vi "$TXXX.vi"(11 "反馈信息":string) -> (3 "接收信息":T1 {"校验和" format="%01xH"; "信息内容"."CRC标志" format="%01xH"; "信息内容"."发信时间分" format="%0d"; "信息内容"."发信时间时" format="%0d"; "信息内容"."信息类别" format="%01xH"})   [LabVIEW 2016, in "BD Protocol 4.0.lvlib" / "BD Protocol 4.0.lvclass"]
uses:
  BD Protocol 4.0.lvclass
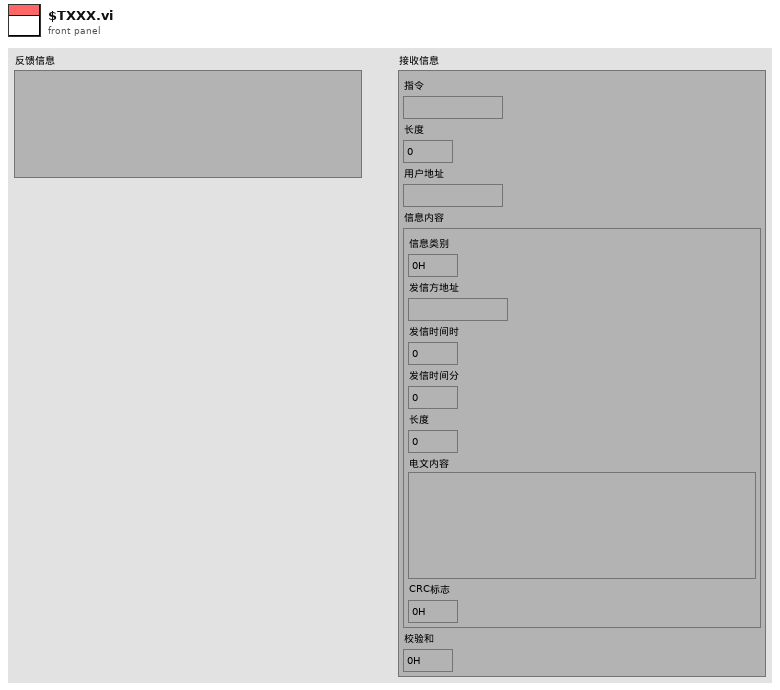
[diagram p1: front panel]
types:
  T1 = cluster{"指令":string, "长度":u16, "用户地址":string, "信息内容":cluster{"信息类别":u8, "发信方地址":string, "发信时间时":u8, "发信时间分":u8, "长度":u16, "电文内容":string, "CRC标志":u8}, "校验和":u8}
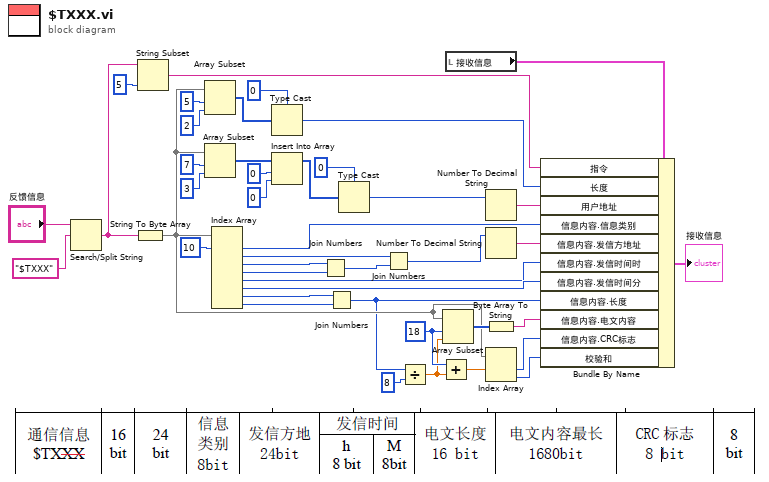
[diagram p0: block diagram]
diagram:
  w12 = 18 ("索引")
  n1 = Search/Split String(string="反馈信息", search string/char (-)="$TXXX" ("搜索字符串/字符(-)")) -> (match + rest of string=w39:string)  [unwired: 1 in, 2 out]
  n2 = String To Byte Array(string=w39) -> (unsigned byte array=w15:u8[])
  n3 = String Subset(string=w39, length (rest)=5 ("长度（剩余）")) -> (substring=w38:string)  [unwired: 1 in]
  n4 = Array Subset(array=w15, index=5 ("索引"), length=2 ("长度")) -> (w35:u8[])
  n5 = Array Subset(array=w15, index=7 ("索引"), length=3 ("长度")) -> (w30:u8[])
  n6 = Index Array(array=w15, index #1=10 ("索引")) -> (element #1=w23:u8, element #2=w18:u8, element #3=w20:u8, element #4=w21:u8, element #5=w4:u8, element #6=w5:u8, element #7=w6:u8, element #8=w7:u8)  [unwired: 7 in]
  n7 = Type Cast(type=u16 0 ("长度"), x=w35) -> (*(type *) &x=w33:u16)
  n8 = Insert Into Array(array=w30, index=0 ("索引"), new element=u8 0 ("新元素/子数组")) -> (w27:u8[])
  n9 = Join Numbers(hi=w20, lo=w21) -> ((hi.lo)=w19:u16)
  n10 = Join Numbers(hi=w6, lo=w7) -> ((hi.lo)=w13:u16)
  n11 = Type Cast(type=u32 0 ("长度"), x=w27) -> (*(type *) &x=w28:u32)
  n12 = Join Numbers(hi=w18, lo=w19) -> ((hi.lo)=w3:u32)
  n13 = Divide(x=w13, y=u16 8) -> (x/y=w8:dbl)
  n14 = Add(x=w12, y=w8) -> (x+y=w14:dbl)
  n15 = Array Subset(array=w15, index=w12, length=w8) -> (w17:u8[])
  n16 = local read "接收信息"() -> (w1:T1)
  n17 = Number To Decimal String(number=w28) -> (decimal integer string=w24:string)  [unwired: 1 in]
  n18 = Number To Decimal String(number=w3) -> (decimal integer string=w2:string)  [unwired: 1 in]
  n19 = Byte Array To String(unsigned byte array=w17) -> (string=w16:string)
  n20 = Index Array(array=w15, index #1=w14) -> (element #1=w11:u8, element #2=w10:u8)  [unwired: 1 in]
  n21 = Bundle By Name(cluster=w1, "指令"=w38, "长度"=w33, "用户地址"=w24, "信息内容.信息类别"=w23, "信息内容.发信方地址"=w2, "信息内容.发信时间时"=w4, "信息内容.发信时间分"=w5, "信息内容.长度"=w13, "信息内容.电文内容"=w16, "信息内容.CRC标志"=w11, "校验和"=w10) -> (→"接收信息":T1)
